vi "play-analyze-z-axis.vi"() -> ()   [LabVIEW 2015]
uses:
  <vilib>/userdefined/High Color/nirio_resource_hc.ctl
  <vilib>/FPGAPlugInAG/cRIO-9082/niLvFpga_Open_cRIO-9082.vi
  <vilib>/rvi/interface/common/dynamic/niFpgaDynamicAddResources.vi
  <vilib>/FPGAPlugInAG/Dynamic/niLvFpga_Reset_Dynamic.vi
  <vilib>/rvi/interface/common/niFpgaWaitOnOcc.vi
  <vilib>/Utility/error.llb/Error Cluster From Error Code.vi
  <vilib>/rvi/errors/niLvFpgaAdjustHostInterfaceError.vi
  <vilib>/FPGAPlugInAG/Dynamic/niLvFpga_Run_Dynamic.vi
  <vilib>/Utility/file.llb/Write To Spreadsheet File (I64).vi
  <vilib>/FPGAPlugInAG/Dynamic/niLvFpga_Close_Dynamic.vi
  <vilib>/rvi/interface/nirviOpenFPGA/nirviOpenFPGA.xnode
  FPGA Bitfiles/afmimagingcontro_FPGATargetSPARTA_analyze-z-axis_yYroOCuDKm4.lvbitx
  <vilib>/rvi/interface/nirviMethod/nirviMethod.xnode
  <vilib>/rvi/interface/nirviReadWriteControl/nirviReadWriteControl.xnode
  <vilib>/rvi/interface/nirviCloseFPGA/nirviCloseFPGA.xnode
  <vilib>/rvi/errors/niLvFpgaMergeErrorWithErrorCode.vi
  <vilib>/FPGAPlugInAG/Dynamic/niLvFpga_ReadFifo_Dynamic.vi
  NiFpgaLv.dll
  <vilib>/rvi/interface/Simulation/niFpgaSimulationCallBeginRW.vi
  <vilib>/FPGAPlugInAG/Dynamic/niLvFpga_ConfigureFifo_Dynamic.vi
panel:
  out "currentCase":i16
  out "caseiter":i16
  in  "trigger-0":bool
  out "Mod2/AI2":fxp<+/-,24,5>
  out "STOP":bool
  out "u(k)":sgl
  in  "init Z up":sgl
  in  "ramp-rate":sgl=-5e-06
  in  "initial-case":u8
  in  "Ki":sgl=0.001
  in  "setpoint":sgl
  in  "nsamps":i32
  out "Waveform Graph":dbl[](graph)
  in  "outputData BOTH":path=path "C:/Users/arnold/Documents/labview/afm_imaging/data/analyze-z-axis-PIon.csv"
  out "y iter":i32
  out "size(s)":i32
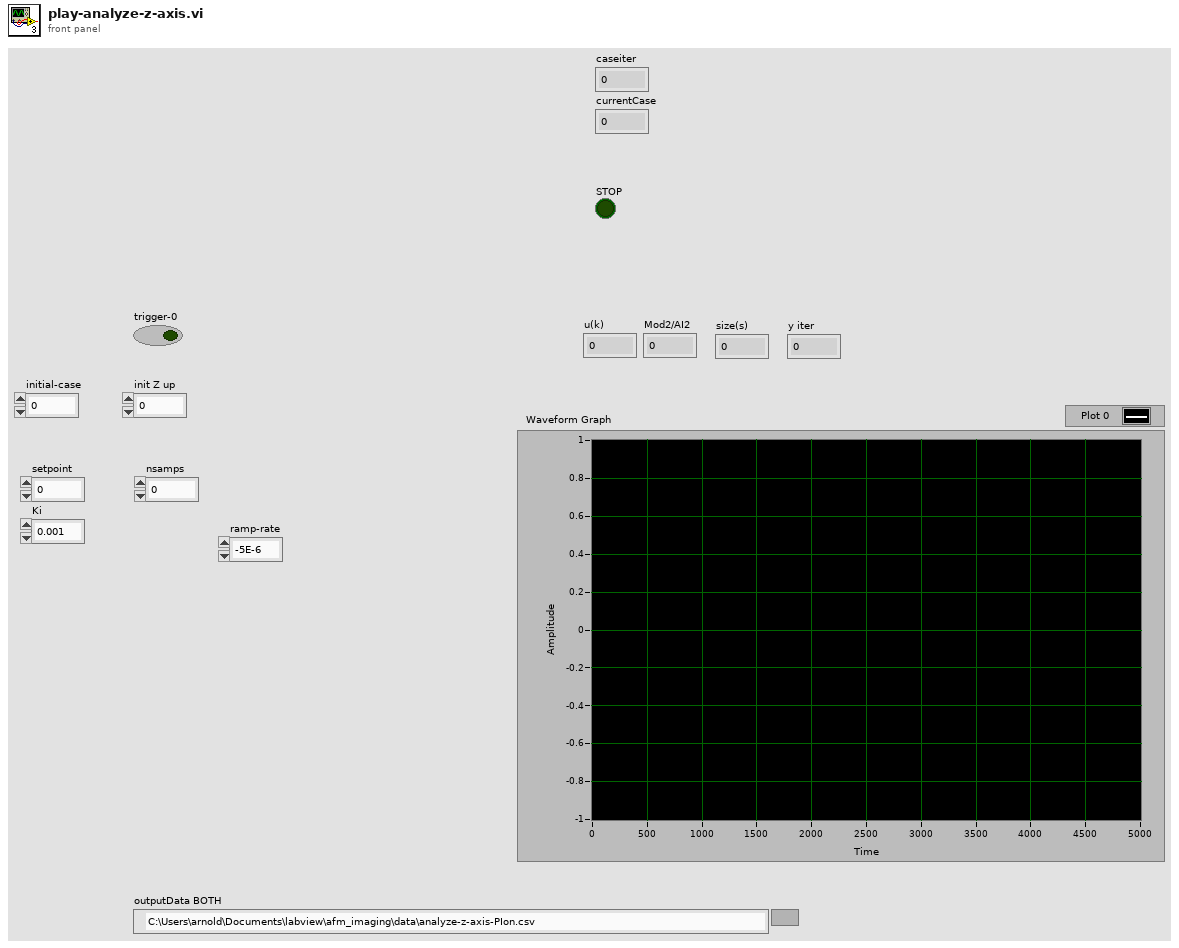
[diagram p1: front panel]
types:
  T1 = typedef "nirio_resource_hc.ctl" = tag
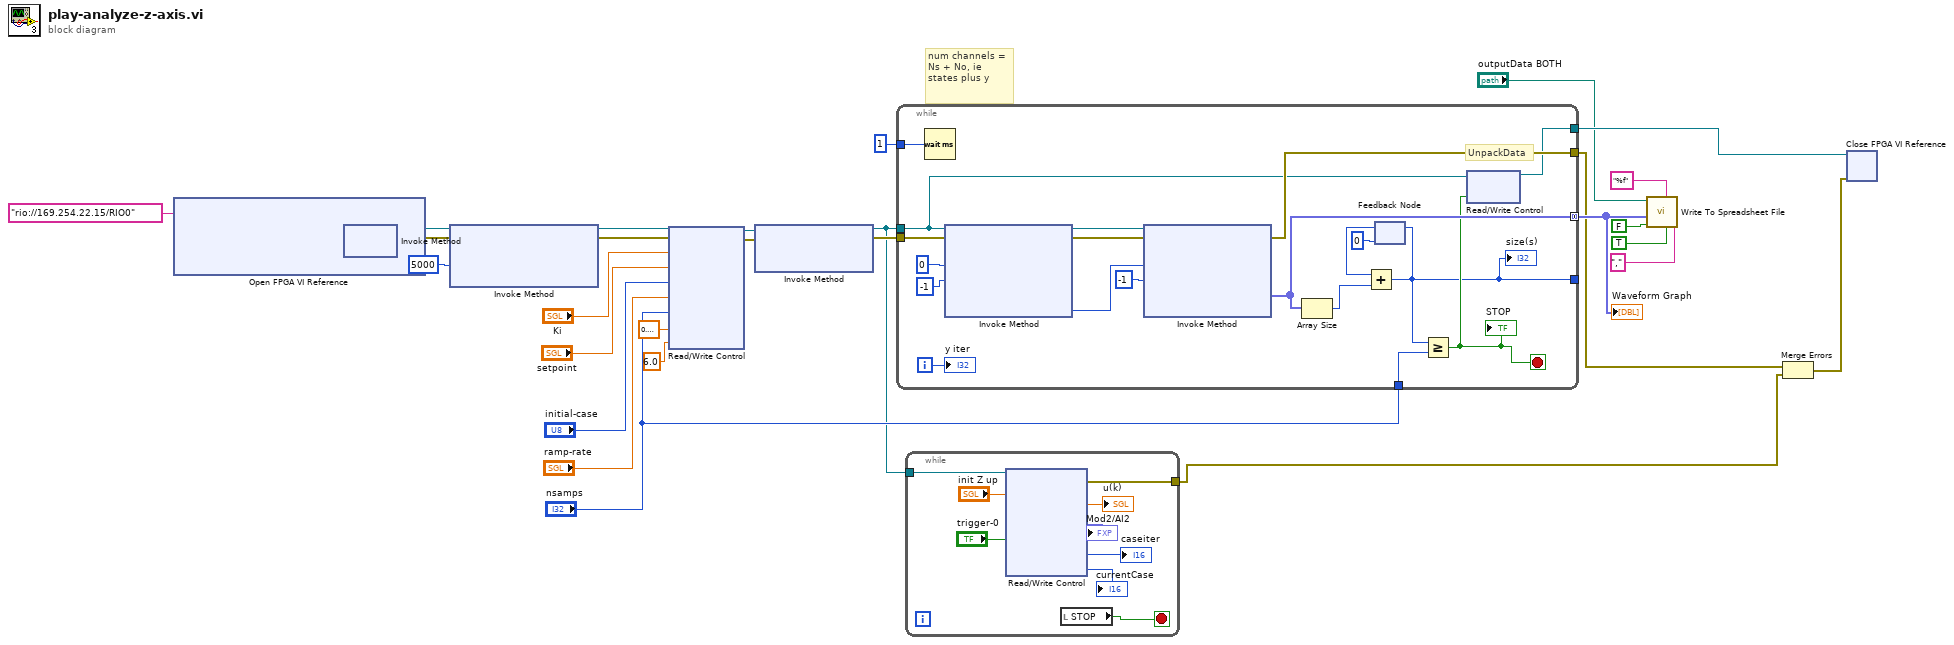
[diagram p0: block diagram]
diagram:
  # "num channels = Ns + No, ie states plus y"
  n1 = xnode "Open FPGA VI Reference"("resource name"=T1 "rio://169.254.22.15/RIO0") -> ("FPGA VI Reference Out"=w27:refnum<k20>, "error out"=w26:errorcluster)  [unwired: 1 in]
  n2 = xnode "Invoke Method"("FPGA VI Reference In"=w27, "error in"=w26) -> ("FPGA VI Reference Out"=w18:refnum<k20>, "error out"=w17:errorcluster)
  n3 = xnode "Invoke Method"("FPGA VI Reference In"=w18, "error in"=w17, "Requested Depth"=5000) -> ("FPGA VI Reference Out"=w15:refnum<k20>, "error out"=w14:errorcluster)  [unwired: 1 out]
  n4 = xnode "Read/Write Control"("FPGA VI Reference In"=w15, "error in"=w14, "Ki"="Ki", "setpoint"="setpoint", "initial-case"="initial-case", "ramp-rate"="ramp-rate", "numIters"="nsamps", "TOL"=sgl 0.3, "uz-max"=sgl 6.0) -> ("FPGA VI Reference Out"=w12:refnum<k20>, "error out"=w13:errorcluster)
  n5 = xnode "Invoke Method"("FPGA VI Reference In"=w12, "error in"=w13) -> ("FPGA VI Reference Out"=w6:refnum<k20>, "error out"=w19:errorcluster)  [unwired: 1 in]
  n6 = while {
    tunnel: 1 -> [w49]
    tunnel: w6 -> [w41]
    tunnel: w19 -> [w35]
    tunnel: [w42] -> w2
    tunnel: [w34] -> w29
    tunnel: [w38] -> w16 mode=concatenating
    tunnel: [w31] -> _
    tunnel: "nsamps" -> [w32]
    i -> [w40]
    stop <- w33 stop-if-true
    # "UnpackData"
    n7 = Wait (ms)(milliseconds to wait=w49) -> ()  [unwired: 1 out]
    n8 = xnode "Invoke Method"("FPGA VI Reference In"=w41, "error in"=w35, "Number of Elements"=0 ("Timeout (ms)"), "Timeout (ms)"=-1) -> ("FPGA VI Reference Out"=w45:refnum<k20>, "error out"=w46:errorcluster, "Elements Remaining"=w39:u32)  [unwired: 1 out]
    n9 = xnode "Invoke Method"("FPGA VI Reference In"=w45, "error in"=w46, "Number of Elements"=w39, "Timeout (ms)"=-1) -> ("error out"=w42:errorcluster, "Data"=w38:fxp<+/-,16,5>[])  [unwired: 2 out]
    n10 = Array Size(array=w38) -> (size(s)=w37:i32)
    n11 = feedback #1(0) -> (w36:i32)
    n12 = Add(x=w36, y=w37) -> (x+y=w31:i32)
    "size(s)" <- w31
    n13 = feedback-in #1(w31) -> ()
    n14 = Greater Or Equal?(x=w31, y=w32) -> (x >= y?=w33:bool)
    "STOP" <- w33
    n15 = xnode "Read/Write Control"("FPGA VI Reference In"=w41, "stop"=w33) -> ("FPGA VI Reference Out"=w34:refnum<k20>)  [unwired: 1 in, 1 out]
    "y iter" <- w40
  }
  "Waveform Graph" <- w16
  n16 = while {
    tunnel: w6 -> [w58]
    tunnel: [w53] -> w3
    stop <- w55 stop-if-true
    n17 = xnode "Read/Write Control"("FPGA VI Reference In"=w58, "init Z up"="init Z up", "trigger-0"="trigger-0") -> ("error out"=w53:errorcluster, "u(k)"=→"u(k)":sgl, "Mod2/AI2"=→"Mod2/AI2":fxp<+/-,24,5>, "caseiter"=→"caseiter":i16, "currentCase"=→"currentCase":i16)  [unwired: 1 in, 1 out]
    n18 = local read "STOP"() -> (w55:bool)
  }
  n19 = call-poly <vilib>:"Write To Spreadsheet File.vi"("delimiter (\\t)"=",", "transpose? (no:F)"=TRUE, "format (%d)"="%f", "append to file? (new file:F)"=FALSE, "1D data"=w16, "file path (dialog if empty)"="outputData BOTH") -> ()  [unwired: 2 in, 1 out]
  n20 = Merge Errors(w2, w3) -> (w1:errorcluster)
  n21 = xnode "Close FPGA VI Reference"("FPGA VI Reference In"=w29, "error in"=w1) -> ()  [unwired: 1 out]
